vi "TestExec.Config, Get Station Name.vi"(11 "App Name":string="Station") -> (1 "App PN Out":string, 3 "App Name Out":string)   [LabVIEW 2018]
uses:
  <vilib>/Utility/config.llb/Read Key (String).vi
  <vilib>/Utility/config.llb/NI_LVConfig.lvlib
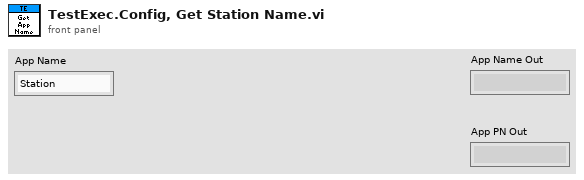
[diagram p1: front panel]
types:
  T1 = enum32{"invalid app kind", "Development System", "Run Time System", "Student Edition", "Embedded LabVIEW", "Evaluation", "Custom"}
  T2 = typedef "NI_LVConfig.lvlib/Config Data RefNum.ctl" = refnum<k1>
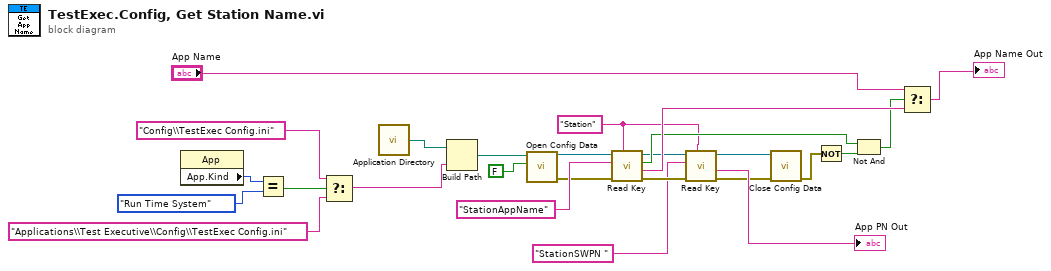
[diagram p0: block diagram]
diagram:
  w7 = "Station" ("section")
  n1 = property class="App"() -> ("App.Kind"=w13:T1)  [unwired: 2 in, 2 out]
  n2 = Equal?(x=w13, y=T1."Run Time System" ("Application:Kind")) -> (x = y?=w9:bool)
  n3 = Select(t="Config\\TestExec Config.ini", s=w9, f="Applications\\Test Executive\\Config\\TestExec Config.ini") -> (s? t:f=w8:string)
  n4 = call <vilib>:"Application Directory.vi"() -> ("Application Directory"=w15:path)
  n5 = Build Path(base path=w15, name or relative path=w8) -> (appended path=w14:path)
  n6 = call <vilib>:"Open Config Data.vi"("create file if necessary (T)"=FALSE, "configuration file path"=w14) -> ("error out"=w24:errorcluster, "refnum"=w26:T2)  [unwired: 7 in, 1 out]
  n7 = call-poly <vilib>:"Read Key.vi"("section"=w7, "error in (no error)"=w24, "key"="StationAppName", "refnum"=w26) -> ("error out"=w3:errorcluster, "value"=w20:string, "found?"=w17:bool, "refnum out"=w2:T2)  [unwired: 4 in]
  n8 = call-poly <vilib>:"Read Key.vi"("section"=w7, "error in (no error)"=w3, "key"="StationSWPN ", "refnum"=w2) -> ("error out"=w4:errorcluster, "value"=→"App PN Out":string, "refnum out"=w5:T2)  [unwired: 4 in, 1 out]
  n9 = call <vilib>:"Close Config Data.vi"("error in (no error)"=w4, "refnum"=w5) -> ("error out"=w18:errorcluster)  [unwired: 8 in, 1 out]
  n10 = Not(x=w18) -> (.not. x?=w19:bool)
  n11 = Not And(1:w19, 2:w17) -> (0:w16:bool)
  n12 = Select(t="App Name", s=w16, f=w20) -> (s? t:f=→"App Name Out":string)
